vi "First Step.vi"(8 "error in (no error)":errorcluster, 11 "Analog Out Scan.lvclass in":refnum<class "Analog Output Scan.lvclass">) -> (0 "error out":errorcluster, 2 "Current Position":dbl, 3 "Analog Out Scan.lvclass out":refnum<class "Analog Output Scan.lvclass">)   [LabVIEW 2017, in "Analog Output Scan.lvclass"]
doc: "(Dynamic) Reset the instrument and prepare to scan. Go to step #0 - the first step. If desired, the scanner may do this in a different way than usual (i.e. by preparing to move a long distance, or reset to home position.)"
uses:
  Analog Output Scan.lvclass
  Analog Output Scan.lvclass/Analog Output Scan.ctl
  <vilib>/DAQmx/write.llb/DAQmx Write (Analog DBL 1Chan 1Samp).vi
  <vilib>/DAQmx/miscellaneous.llb/DAQmx Fill In Error Info.vi
  Scanner/Scanner.lvclass
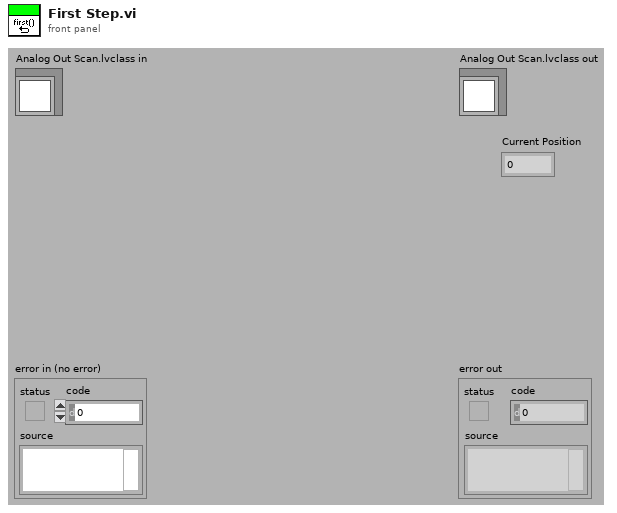
[diagram p1: front panel]
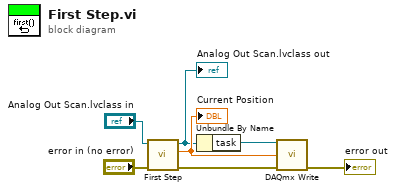
[diagram p0: block diagram]
diagram:
  n1 = call-parent "First Step.vi"("error in (no error)"="error in (no error)", "Scanner.lvclass in"="Analog Out Scan.lvclass in") -> ("error out"=w1:errorcluster, "Current Position"=w4:dbl, "Scanner.lvclass out"=w3:refnum<class "Analog Output Scan.lvclass">)  [unwired: 7 in]
  "Analog Out Scan.lvclass out" <- w3
  "Current Position" <- w4
  n2 = Unbundle By Name(w3) -> ("task"=w2:refnum<k21>)
  n3 = call-poly <vilib>:"DAQmx Write.vi"("task/channels in"=w2, "data"=w4, "error in"=w1) -> ("error out"=→"error out":errorcluster)  [unwired: 10 in, 2 out]
